vi "Write Pct_of_X.vi"(8 "error in (no error)":errorcluster, 10 "Pct_of_X?":bool, 11 "AssertEqualValue in":refnum<class "AssertAlmostEqualValue.lvclass">) -> (0 "error out":errorcluster, 3 "AssertEqualValue out":refnum<class "AssertAlmostEqualValue.lvclass">)   [LabVIEW 2021, in "Bananas.lvlib" / "AssertAlmostEqualValue.lvclass"]
uses:
  AssertAlmostEqualValue.lvclass
  AssertAlmostEqualValue.lvclass/AssertAlmostEqualValue.ctl
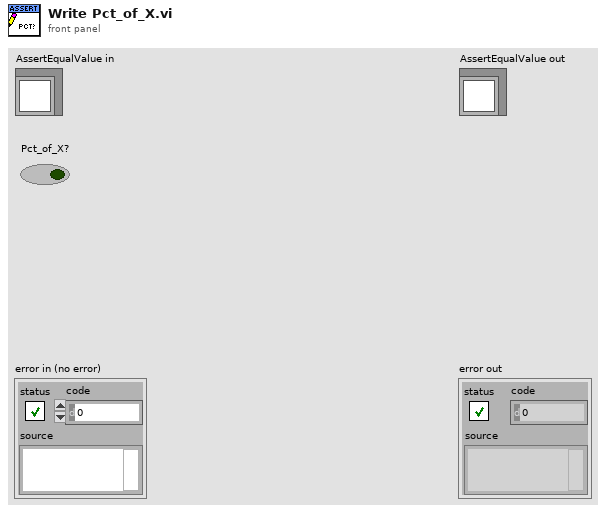
[diagram p1: front panel]
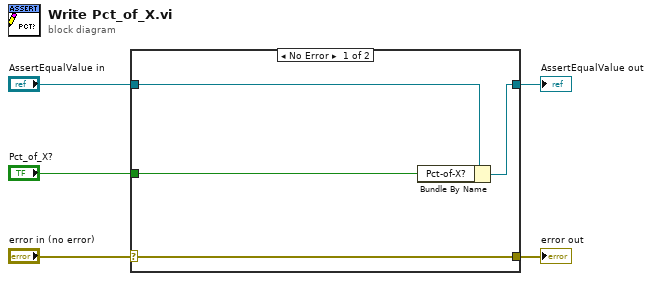
[diagram p0: block diagram]
diagram:
  n1 = case shown="No Error" "error in (no error)" {
    selector: "error in (no error)" -> [w9 w10]
    tunnel: [w9 w10] -> w4
    tunnel: [w7 w11] -> w2
    tunnel: "AssertEqualValue in" -> [w8 w11]
    tunnel: "Pct_of_X?" -> [w6 _]
    frame No Error {
      n2 = Bundle By Name(cluster=w8, "Pct-of-X?"=w6) -> (w7:refnum<class "AssertAlmostEqualValue.lvclass">)
    }
    frame Error {
    }
  }
  "error out" <- w4
  "AssertEqualValue out" <- w2
